vi "TX OOB Test Cases.vi"() -> (0 "error out":errorcluster, 2 "status":string, 3 "pass":bool)   [LabVIEW 2021]
uses:
  CIFUtilities/CIFOutOfBand/CIFOutOfBand.lvclass/CIFOutOfBand.ctl
  OOB_Rx/Typedef/OOB Commands.ctl
  OOB_Tx/Private/Command Settings.vi
  CIFUtilities/CIFOutOfBand/Accessors/Write Local OOB Data.vi
  CIFUtilities/CIFOutOfBand/Accessors/Read Local OOB Data.vi
  CIFUtilities/CIFOutOfBand/Write OOB DVR.vi
  CIFUtilities/CIFOutOfBand/Utilities/Command to Bitwise Command.vi
  CIFUtilities/CIFOutOfBand/Read OOB DVR.vi
  OOB_Tx/Private/Read Payload.vi
  OOB_Tx/CIFCustomOOB_Tx.lvclass
  D:/dev/CIF-LVCore/src/CIFUtilities/CIFOutOfBand/CIFOutOfBand.lvclass
  CIFUtilities/CIFOutOfBand/Init OOB.vi
  CIFUtilities/CIFOutOfBand/CIFOutOfBand.lvclass
  OOB_Rx/CIFTCustomOOB_Rx.lvclass
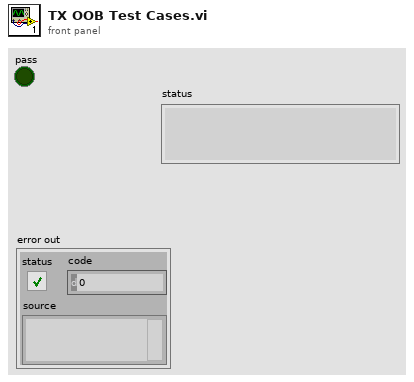
[diagram p1: front panel]
types:
  T1 = typedef "CIFTCustomOOB_Rx.lvclass/OOB Commands.ctl" = enum8{"Update Data"}
  T2 = typedef "CIFCustomOOB_Tx.lvclass/OOB Commands.ctl" = enum8{"Update Data"}
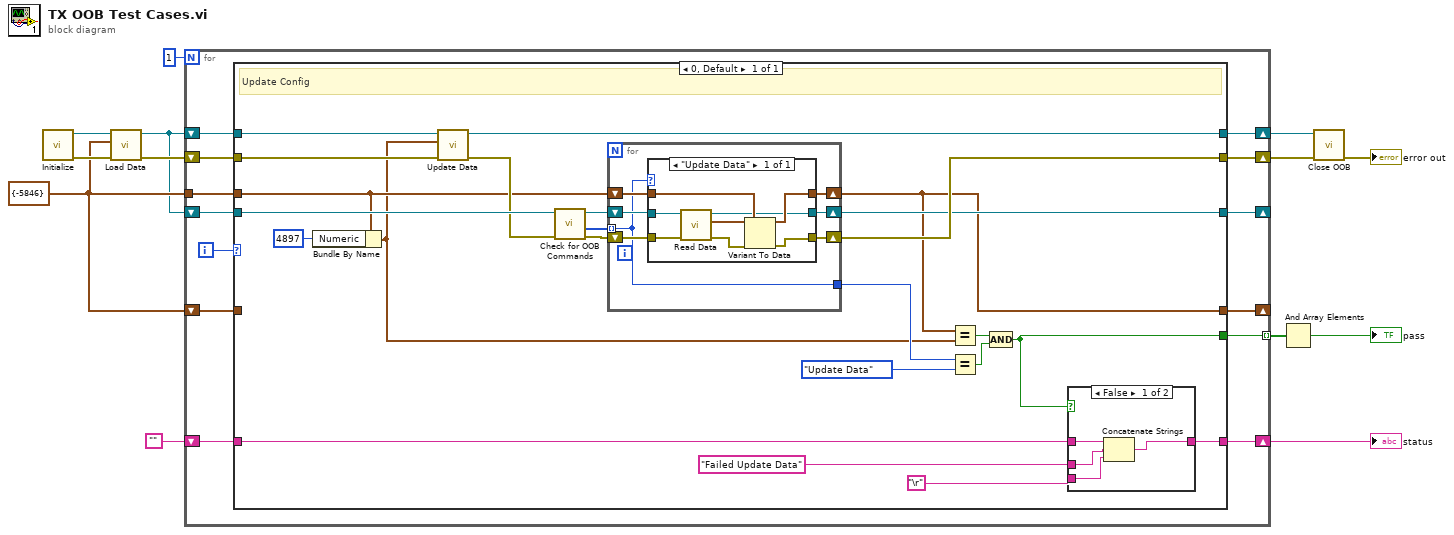
[diagram p0: block diagram]
diagram:
  w2 = cluster{"Numeric":i32} {"Numeric"=-5846} ("Data")
  n1 = call "Initialize.vi"() -> ("error out"=w7:errorcluster, "CutomOOB_Tx out"=w6:refnum<class "CIFCustomOOB_Tx.lvclass">)  [unwired: 10 in]
  n2 = call "Load Data.vi"("error in (no error)"=w7, "Data"=w2, "CutomOOB_Tx in"=w6) -> ("error out"=w5:errorcluster, "CutomOOB_Tx out"=w1:refnum<class "CIFCustomOOB_Tx.lvclass">)  [unwired: 7 in]
  n3 = for {
    N: 1 -> [_]
    tunnel: [w26] -> w11 mode=indexing
    tunnel: w2 -> [w24]
    shift-right: [w23] -> w12
    shift-left: w5 -> [w25]
    shift-right: [w14] -> w13
    shift-left: w1 -> [w15]
    shift-right: [w20] -> _
    shift-left: w1 -> [w21]
    shift-right: [w19] -> _
    shift-left: w2 -> [w18]
    shift-right: [w16] -> w8
    shift-left: "" -> [w17]
    i -> [w22]
    n4 = case shown="0, Default" w22 {
      tunnel: [w37] -> w26
      tunnel: w25 -> [w33]
      tunnel: w24 -> [w31]
      tunnel: w15 -> [w29]
      tunnel: [w49] -> w23
      tunnel: [w34] -> w14
      tunnel: w21 -> [w43]
      tunnel: [w48] -> w20
      tunnel: [w30] -> w19
      tunnel: w18 -> [_]
      tunnel: w17 -> [w47]
      tunnel: [w46] -> w16
      frame 0, Default {
        # "Update Config"
        n5 = Bundle By Name(cluster=w31, "Numeric"=4897) -> (w27:cluster{"Numeric":i32})
        n6 = call "Update Data.vi"("error in"=w33, "Data"=w27, "CutomOOB_Tx in"=w29) -> ("error out"=w32:errorcluster, "CutomOOB_Tx out"=w34:refnum<class "CIFCustomOOB_Tx.lvclass">)  [unwired: 7 in]
        n7 = call "Check for OOB Commands.vi"("error in (no error)"=w32, "CutomOOB_Tx in"=w43) -> ("error out"=w42:errorcluster, "Commands"=w40:T2[], "CutomOOB_Tx out"=w41:refnum<class "CIFCustomOOB_Tx.lvclass">)  [unwired: 6 in, 1 out]
        n8 = for {
          tunnel: w40 -> [w50] mode=indexing
          shift-right: [w51] -> w30
          shift-left: w31 -> [w56]
          shift-right: [w55] -> w49
          shift-left: w42 -> [w53]
          shift-right: [w54] -> w48
          shift-left: w41 -> [w52]
          tunnel: [w50] -> w36
          n9 = case shown="\"Update Data\"" w50 {
            tunnel: w52 -> [w60]
            tunnel: w53 -> [w61]
            tunnel: [w59] -> w54
            tunnel: w56 -> [w64]
            tunnel: [w63] -> w55
            tunnel: [w62] -> w51
            frame "Update Data" {
              n10 = call "Read Data.vi"("error in"=w61, "CutomOOB_Tx in"=w60) -> ("error out"=w57:errorcluster, "Data"=w58:cluster{"Numeric":i32}, "CutomOOB_Tx out"=w59:refnum<class "CIFCustomOOB_Tx.lvclass">)  [unwired: 7 in]
              n11 = Variant To Data(error in=w57, type=w64, Variant=w58) -> (data=w62:cluster{"Numeric":i32}, error out=w63:errorcluster)
            }
          }
        }
        n12 = Equal?(x=w30, y=w27) -> (x = y?=w39:bool)
        n13 = Equal?(x=w36, y=OOB_Commands."Update Data") -> (x = y?=w38:bool)
        n14 = Compound Arithmetic op=AND(w39, w38) -> (w37:bool)
        n15 = case shown="False" w37 {
          tunnel: w47 -> [w68 w69]
          tunnel: [w65 w69] -> w46
          tunnel: "Failed Update Data" -> [w67 _]
          tunnel: "\r" -> [w66 _]
          frame False {
            n16 = Concatenate Strings(w68, w67, w66) -> (w65:string)
          }
          frame True {
          }
        }
      }
    }
  }
  "status" <- w8
  n17 = And Array Elements(Boolean array=w11) -> (logical AND=→"pass":bool)
  n18 = call "Close OOB.vi"("error in"=w12, "OOB in"=w13) -> ("error out"=→"error out":errorcluster)  [unwired: 9 in]
